vi "WHD_VEten_0.1_WS_BIDIREC_Pruebas.vi"() -> ()   [LabVIEW 2015]
uses:
  <vilib>/NI_Real-Time Target Support.lvlib
  <vilib>/rvi/interface/nirviReadWriteControl/nirviReadWriteControl.xnode
  <vilib>/rvi/interface/nirviMethod/nirviMethod.xnode
  <vilib>/rvi/interface/nirviOpenFPGA/nirviOpenFPGA.xnode
  <vilib>/rvi/interface/nirviCloseFPGA/nirviCloseFPGA.xnode
  <vilib>/userdefined/High Color/nirio_resource_hc.ctl
  <vilib>/Utility/file.llb/Write To Spreadsheet File (string).vi
  AURA_Wheel/Json2Labv.lvlib
  AURA_Wheel/AuraWheelAPI/AuraWheel.lvlib
  <vilib>/LabVIEW Targets/FPGA/cRIO/shared/nicrio_ModuleControls/nicrio_cRIO-9234_DataRatesRing2.ctl
  NiFpgaLv.dll
  <vilib>/Utility/error.llb/Error Cluster From Error Code.vi
  <vilib>/rvi/errors/niLvFpgaAdjustHostInterfaceError.vi
  <vilib>/rvi/errors/niLvFpgaMergeErrorWithErrorCode.vi
  <vilib>/Utility/file.llb/Write Delimited Spreadsheet (string).vi
  FPGA Bitfiles/W&RDEuskotrenIBA_FPGATarget2_FPGA8a2wsBIdirec_MwruJOs6jio.lvbitx
  <vilib>/FPGAPlugInAG/cRIO-9031/niLvFpga_Close_cRIO-9031.vi
  <vilib>/FPGAPlugInAG/cRIO-9031/niLvFpga_Open_cRIO-9031.vi
  <vilib>/FPGAPlugInAG/cRIO-9031/niLvFpga_Run_cRIO-9031.vi
  <vilib>/FPGAPlugInAG/cRIO-9031/niLvFpga_ConfigureFifo_cRIO-9031.vi
  <vilib>/FPGAPlugInAG/cRIO-9031/niLvFpga_StartFifo_cRIO-9031.vi
  <vilib>/FPGAPlugInAG/cRIO-9031/niLvFpga_ReadFifo_cRIO-9031.vi
  <vilib>/FPGAPlugInAG/cRIO-9031/niLvFpga_StopFifo_cRIO-9031.vi
  <vilib>/FPGAPlugInAG/cRIO-9031/niLvFpga_Reset_cRIO-9031.vi
panel:
  out "TAGs_AURAwheel":string[][](array[string])
  out "Plataformas?":bool
  out "Ejes_convoy":i32
  out "Nº Ejes":i32[](array[numeric])
  out "Nº UTs":i32
  out "it-read-LR6":i32[](array[numeric])
  out "it-LR6":i32
  out "RFID_LR6_Error":errorcluster
  out "TAGs HEX":string[](array[string])
  out "TAGs LR6":string[](array[string])
  in  "TAGs HEX 2":string[](array[string])
  out "Series_flota":string[](array[string])
  out "Tabla_flota":string[][](array[string])
  out "Puntos medios de las ventanas":dbl[][](array[numeric])
  in  "User":string
  in  "Índice de los archivos seleccionados":i32
  in  "Array":path[][](array[path])=[[path "c:/Trenes_prueba/0207_2013-09-24_19-09-42_0.bin", path "c:/Trenes_prueba/0096_2013-10-30_18-13-14_0.bin", path "c:/Trenes_prueba/0001_2013-06-05_13-06-23_0.bin"], [path "c:/Trenes_prueba/0207_2013-09-24_19-09-42_1.bin", path "c:/Trenes_prueba/0096_2013-10-30_18-13-14_1.bin", path "c:/Trenes_prueba/0001_2013-06-05_13-06-23_1.bin"], [path "c:/Trenes_prueba/0207_2013-09-24_19-09-42_2.bin", path "c:/Trenes_prueba/0096_2013-10-30_18-13-14_2.bin", path "c:/Trenes_prueba/0001_2013-06-05_13-06-23_2.bin"], [path "c:/Trenes_prueba/0207_2013-09-24_19-09-42_3.bin", path "c:/Trenes_prueba/0096_2013-10-30_18-13-14_3.bin", path "c:/Trenes_prueba/0001_2013-06-05_13-06-23_3.bin"], [path "c:/Trenes_prueba/0207_2013-09-24_19-09-42_4.bin", path "c:/Trenes_prueba/0096_2013-10-30_18-13-14_4.bin", path "c:/Trenes_prueba/0001_2013-06-05_13-06-23_4.bin"], [path "c:/Trenes_prueba/0207_2013-09-24_19-09-42_5.bin", path "c:/Trenes_prueba/0096_2013-10-30_18-13-14_5.bin", path "c:/Trenes_prueba/0001_2013-06-05_13-06-23_5.bin"], [path "c:/Trenes_prueba/0207_2013-09-24_19-09-42_6.bin", path "c:/Trenes_prueba/0096_2013-10-30_18-13-14_6.bin", path "c:/Trenes_prueba/0001_2013-06-05_13-06-23_6.bin"], [path "c:/Trenes_prueba/0207_2013-09-24_19-09-42_7.bin", path "c:/Trenes_prueba/0096_2013-10-30_18-13-14_7.bin", path "c:/Trenes_prueba/0001_2013-06-05_13-06-23_7.bin"], [path "c:/Trenes_prueba/0207_2013-09-24_19-09-42_8.bin", path "c:/Trenes_prueba/0096_2013-10-30_18-13-14_8.bin", path "c:/Trenes_prueba/0001_2013-06-05_13-06-23_8.bin"]]
  out "configuration file path":path=path "c:/Parametros.cfg"
  in  "IP synchr":string
  in  "Canal ccero?":bool
  in  "Digital?":bool=TRUE
  out "Numeric 3":i32
  out "data":cluster{"status":string}
  out "confRFID":path=path "c:/RFID/TAGS.csv"
  out "TAGS leidos":path=path "c:/RFID/TAGS.csv"
  in  "Use Aura?":bool
  in  "Parametros AuraWheel":string[](array[string])
  in  "Parámetros acelerómetros":dbl[](array[numeric])
  in  "Number of Samples":u32=5000
  in  "x*y":dbl[](array[numeric])=array[252000 elements]
  out "RFID_Error 2":errorcluster
  in  "milliseconds to wait":u32=180000
  in  "Adquirir continuado":bool
  in  "Tiempo de adquisicion":dbl=10.0
  in  "Adquirir":bool
  in  "Señal digital?":bool=TRUE
  out "Inductivo OK?":bool=TRUE
  out "Acelerómetros OK?":bool[](array[boolean])
  out "Fin":bool
  out "Contador":i32=1
  out "Path TEST":path=path "c:/TEST"
  out "Fallo fotocelula":bool
  out "Path_Borrar":path=path "c:/Trenes"
  out "Longitud de la unidad":dbl
  out "Bucle Espera":i32
  out "Aviso no detección":string
  out "Time to Acquire Block (ms)":i32
  out "Distancia de acelerómetros":dbl[](array[numeric])
  out "Block Size":u32
  out "Distancias generales":dbl[](array[numeric])
  in  "Reset del controlador":bool
  in  "Configuración":bool
  in  "Parar la aplicación":bool
  out "Acel 4":bool=TRUE
  out "Acel 3":bool=TRUE
  out "Acel 2":bool=TRUE
  out "Acel 1":bool=TRUE
  out "RFID":bool=TRUE
  out "date/time string":string
  out "Obstruido?":bool
  out "Tiempo":dbl
  out "Inicio pasada":timestamp
  out "Ultimo TEST":timestamp
  out "Fuente":bool=TRUE
  out "Estado":string
  out "RFID_ID":refnum<k5>
  out "DC OK":string
  out "Aviso temperatura":string
  in  "Tab Control":T1(tab)=enum."Parámetros"
  out "V (m/s)":dbl
  out "Temperatura (ºC)":dbl
  out "Max RMS Ruedas":dbl[][](array[numeric])
  out "result":bool
  out "TAGs":string[](array[string])
  out "Direccion 0?":bool
  out "RuedaDetectada2?":bool=TRUE
  out "RuedaDetectada1?":bool=TRUE
  out "Parar":bool
  out "Waveform Graph":sgl[][](graph)
  out "Nombre de archivo":path[](array[path])
  out "Tiempo de paso (s)":dbl
  out "Tiempo extra de adquisición (s)":dbl
  out "Número de ejes detectados":i32
  out "Buffer Underflow":bool
  out "Buffer Overflow":bool
  out "Disco Duro Disponible (bytes)":i64
  out "created path":path
  out "Nº Ruedas 1":i32
  out "NºRuedas 2":i32
  out "Fallo sensores":string
  out "T fuera rango":bool
  in  "Frecuencia de muestreo (Hz)":dbl=25600.0
  in  "Escaneos de la FIFO por canal":u32=1000
  in  "Tiempo extra al detector de paso (s)":dbl=1.0
  in  "Filtro digital (ms)":u16=13
  in  "dt RMS":dbl=256.0
  in  "Frecuencia de muestreo y módulo CRIO":T2=2 items=["51.200 kS/s (NI 9234)"=1, "25.600 kS/s (NI 9234)"=2, "17.067 kS/s (NI 9234)"=3, "12.800 kS/s (NI 9234)"=4, "10.240 kS/s (NI 9234)"=5, "8.533 kS/s (NI 9234)"=6, "7.314 kS/s (NI 9234)"=7, "6.400 kS/s (NI 9234)"=8, "5.689 kS/s (NI 9234)"=9, "5.120 kS/s (NI 9234)"=10, "4.654 kS/s (NI 9234)"=11, "4.267 kS/s (NI 9234)"=12, "3.938 kS/s (NI 9234)"=13, "3.657 kS/s (NI 9234)"=14, "3.413 kS/s (NI 9234)"=15, "3.200 kS/s (NI 9234)"=16, "3.012 kS/s (NI 9234)"=17, "2.845 kS/s (NI 9234)"=18, "2.695 kS/s (NI 9234)"=19, "2.560 kS/s (NI 9234)"=20, "2.438 kS/s (NI 9234)"=21, "2.328 kS/s (NI 9234)"=22, "2.226 kS/s (NI 9234)"=23, "2.133 kS/s (NI 9234)"=24, "2.048 kS/s (NI 9234)"=25, "1.969 kS/s (NI 9234)"=26, "1.896 kS/s (NI 9234)"=27, "1.829 kS/s (NI 9234)"=28, "1.765 kS/s (NI 9234)"=29, "1.707 kS/s (NI 9234)"=30, "1.652 kS/s (NI 9234)"=31]
  in  "Puerto RFID":u16=2189
  in  "IP RFID":string="192.168.106.99"
  in  "Offset_rueda":fxp<+/-,24,-4>=0.004999998956918716 format="%.27g"
  in  "Count(mSec)":u32=2
  in  "LR6 IP address":string="192.168.106.94"
  in  "Port LR6":u16=2001
  in  "Number of Channels":u32=9
  in  "Pruebas RFID 2":bool
  in  "Pruebas RFID 1":bool
  in  "Descargar":bool
  out "Parámetros":bool=TRUE
  out "Distacias y medidas de dispositivos":bool=TRUE
  out "RFID_Error":errorcluster
  out "error FPGA":errorcluster
  out "error manipulacion archivos":errorcluster
  out "Unidades y ejes":bool=TRUE
  out "RFID":bool=TRUE
  out "error AURA":errorcluster
  out "Response headers":string
  # "Funciona?"
  # "Inductivo"
  # "A4"
  # "A3"
  # "A1"
  # "A2"
  # "WRD_MEX\nWRD_ZAR"
  # "0 tagMexInit\n1 tagMexFin\n\n0 tag1\n1 tag2"
  # "Última detección de unidad"
  # "Error!!"
  # "Estado de la memoria"
  # "Espera"
  # "Adquisicion"
  # "Adquisicion"
  # "Procesado"
  # "Procesado"
  # "Procesado"
  # "Procesado"
  # "Procesado"
  # "Parámetros de muestreo"
  # "Parámetros de adquisición"
  # "Parámetros de procesado"
  # "Cambio Fecha y Hora"
  # "Descarga de planos y TEST"
  # "NO"
  # "SI"
  # "Descarga archivos binarios de adquisición"
  # "NO"
  # "SI"
  # "Cargar datos de configuración"
  # "Errores!!"
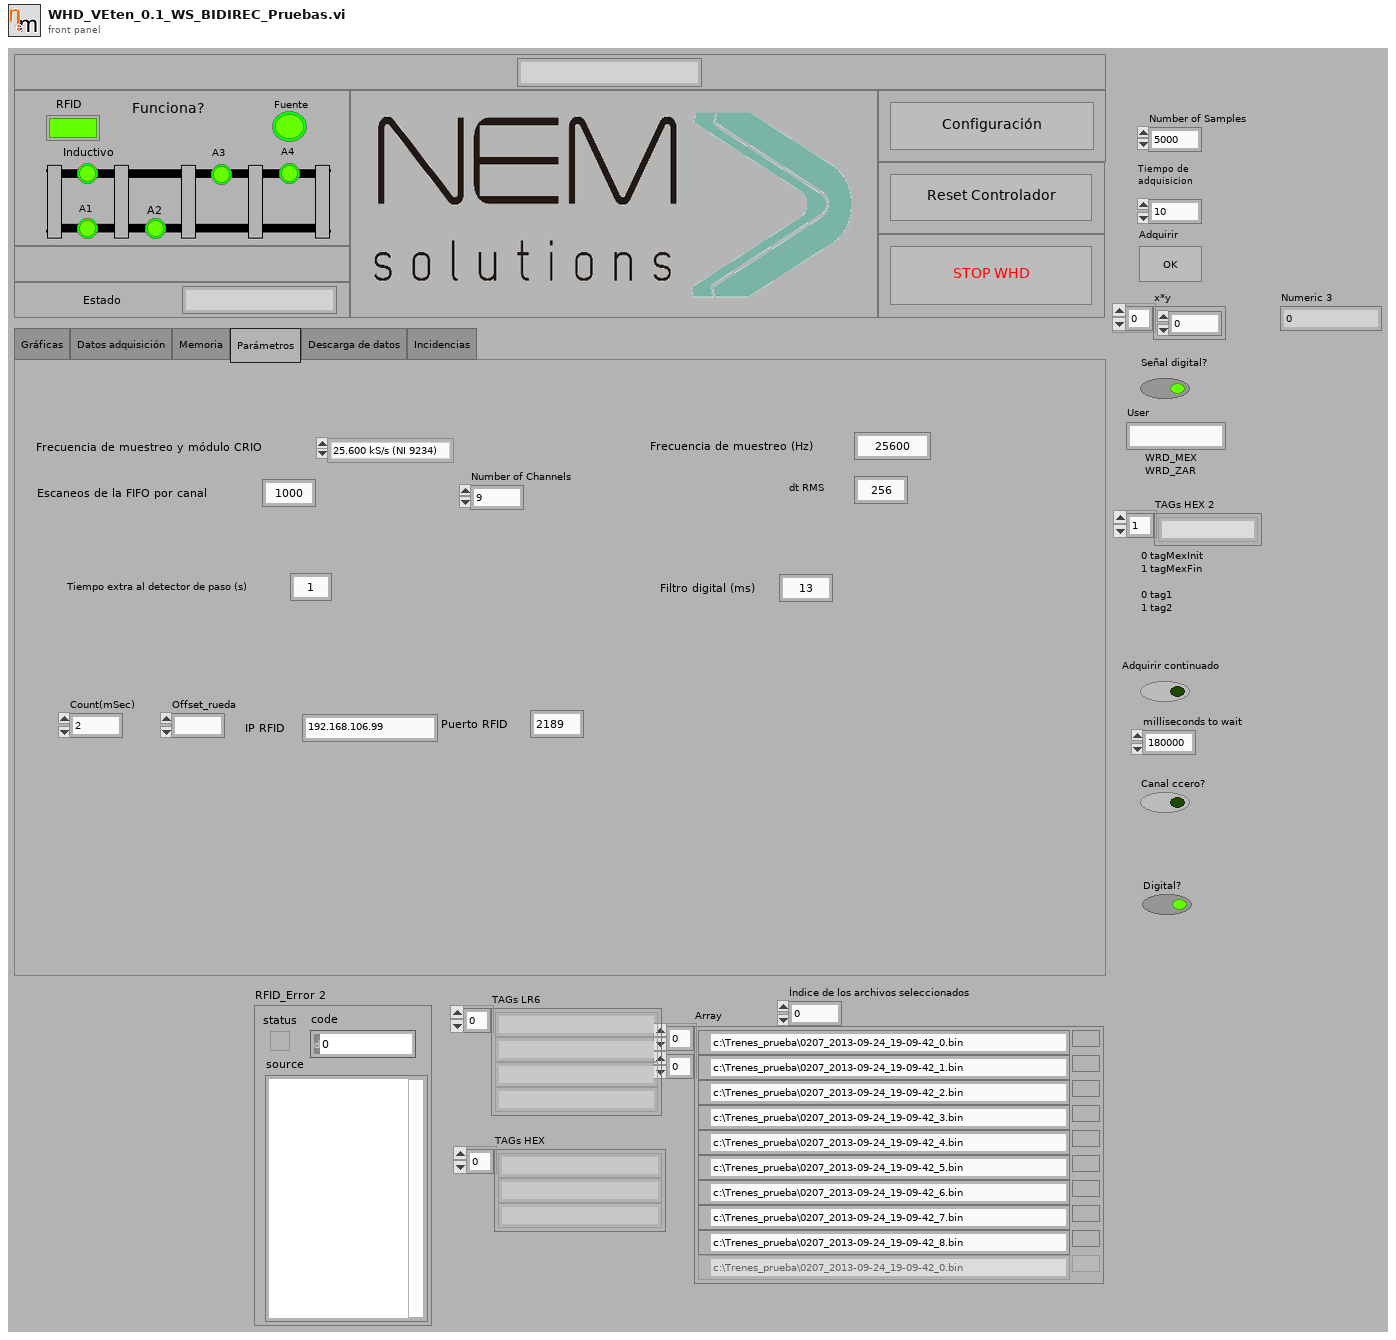
[diagram p1: front panel]
types:
  T1 = enum32{"Gráficas", "Datos adquisición", "Memoria", "Parámetros", "Descarga de datos", "Incidencias"}
  T2 = typedef "nicrio_cRIO-9234_DataRatesRing2.ctl" = u8
  T3 = typedef "nirio_resource_hc.ctl" = tag
  T4 = enum16{"Standard", "Buffered", "CRLF", "Immediate"}
  T5 = enum16{"open", "replace", "create", "open or create", "replace or create", "replace or create with confirmation"}
  T6 = enum16{"big-endian, network order", "native, host order", "little-endian"}
  T7 = cluster{"error IO":errorcluster, bool[], u32[], string[], dbl[]}
  T8 = cluster{"g_ts":dbl, "p_sp":dbl, "p_tp":dbl, "p_tg":cluster{"tg_n":dbl, "tg_t":string}[], "p_ax":cluster{"ax_n":dbl, "ax_sp":dbl, "ax_wh":cluster{"wh_p":dbl, "wh_a1":dbl, "wh_a2":dbl, "wh_a3":dbl, "wh_a4":dbl}[]}[]}
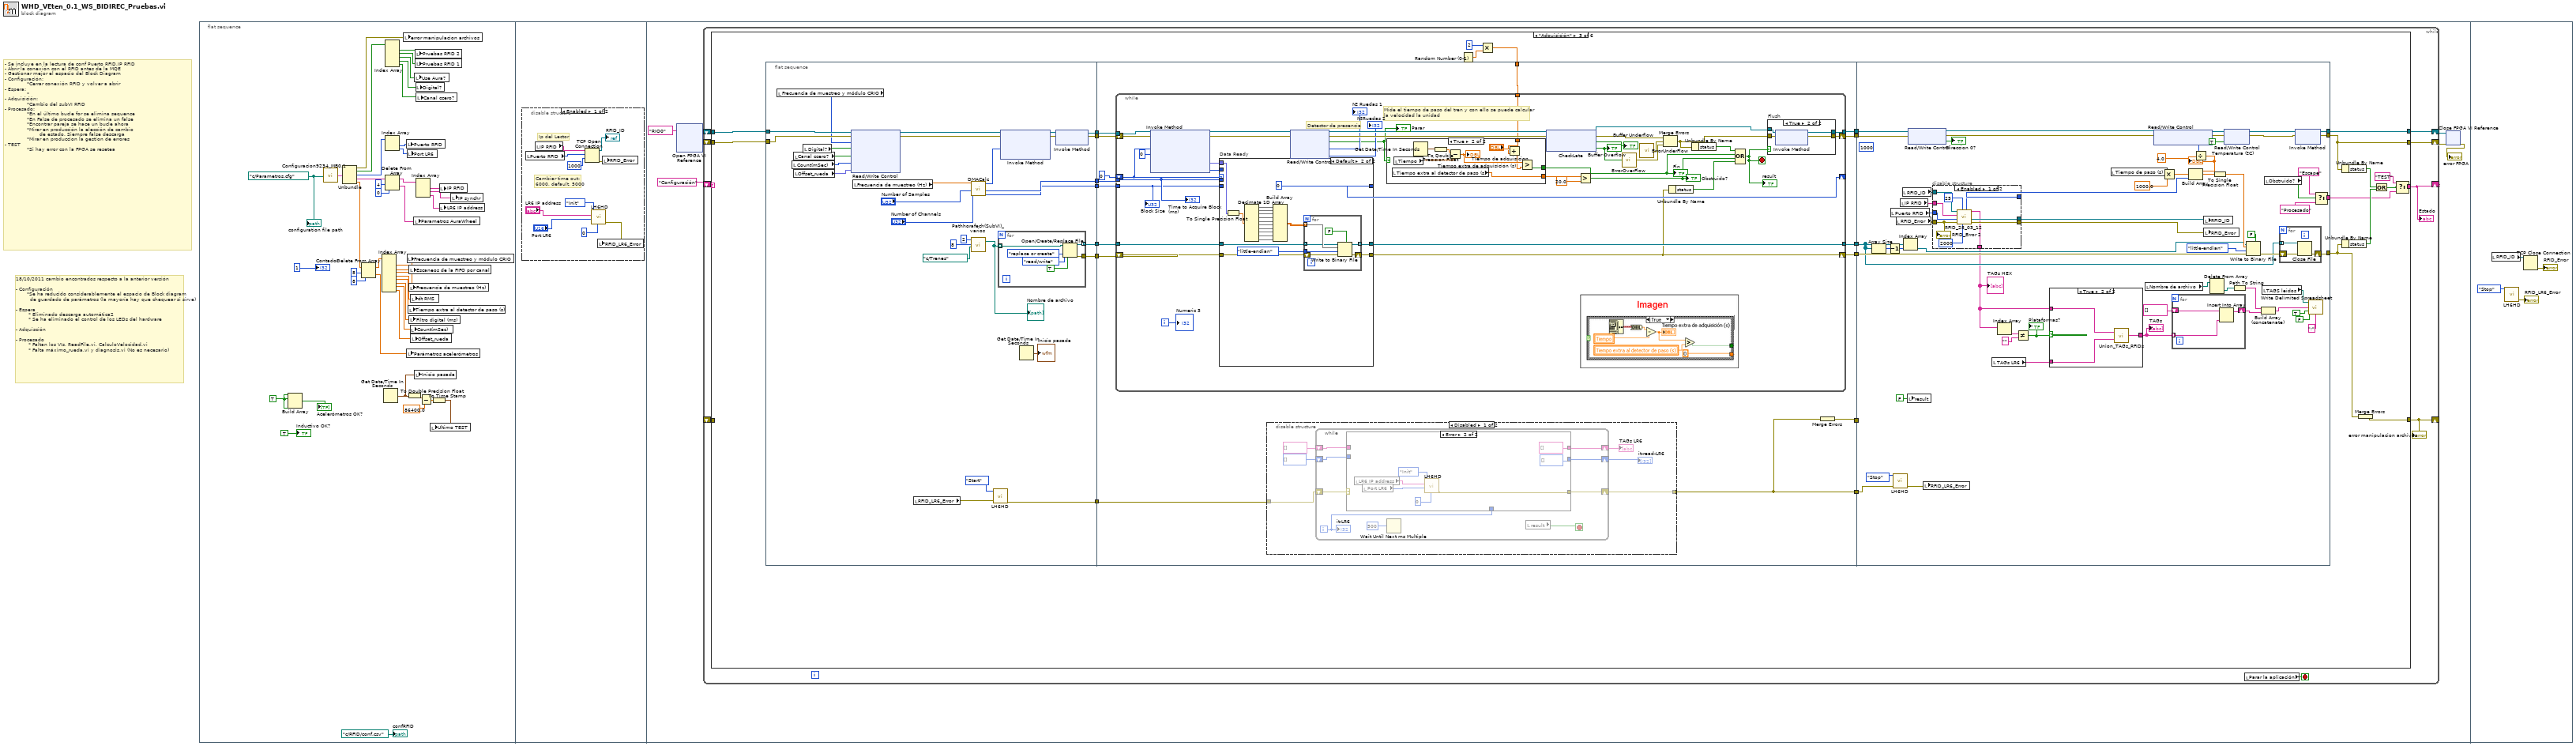
[diagram p0: block diagram]
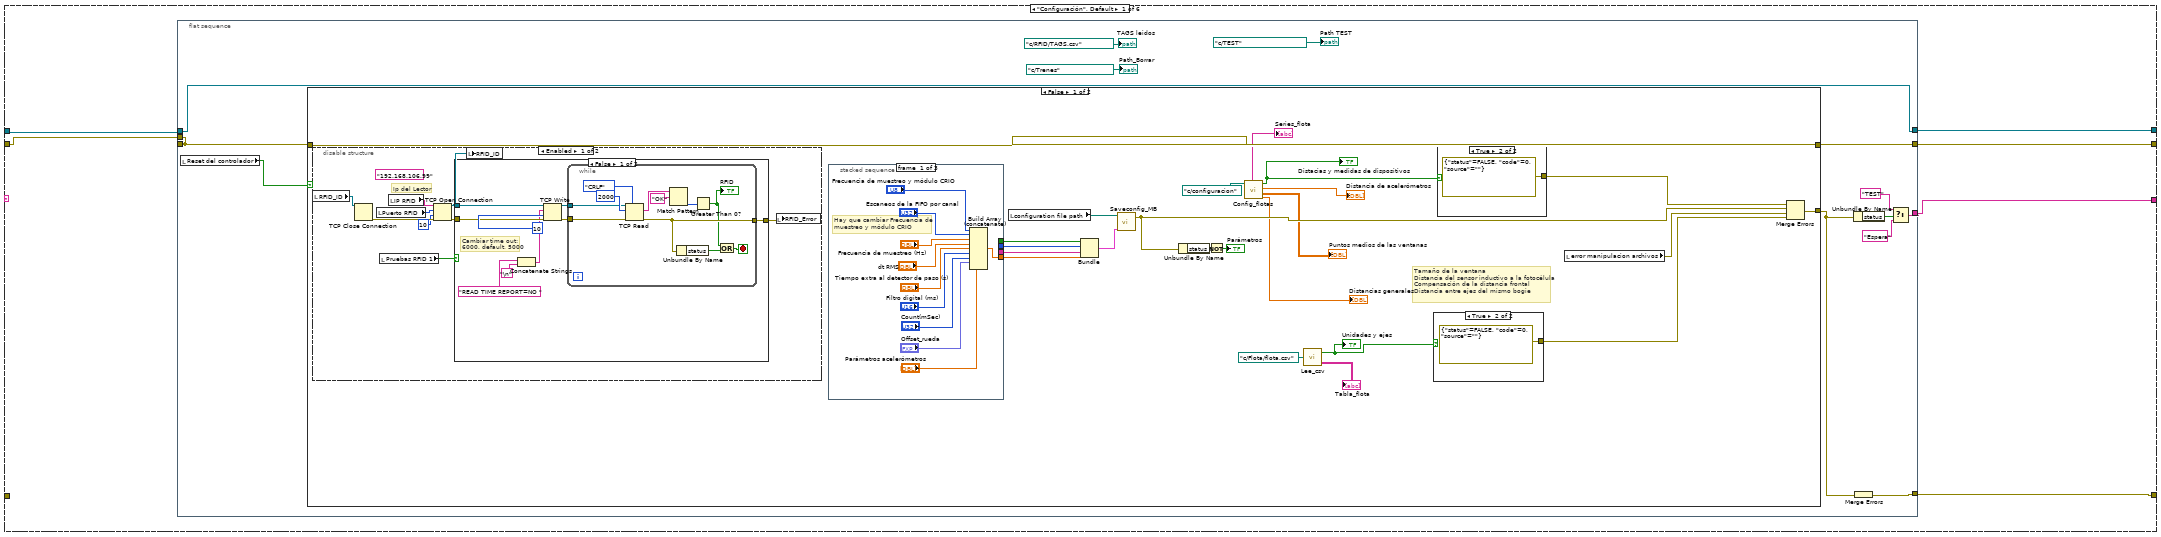
[diagram p3: hidden frame]
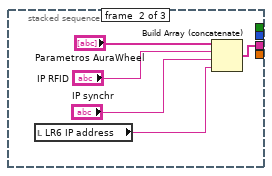
[diagram p4: hidden frame]
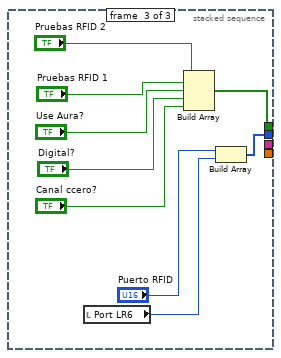
[diagram p5: hidden frame]
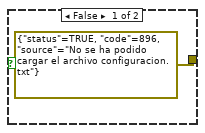
[diagram p6: hidden frame]
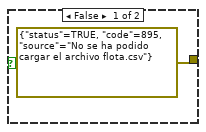
[diagram p7: hidden frame]
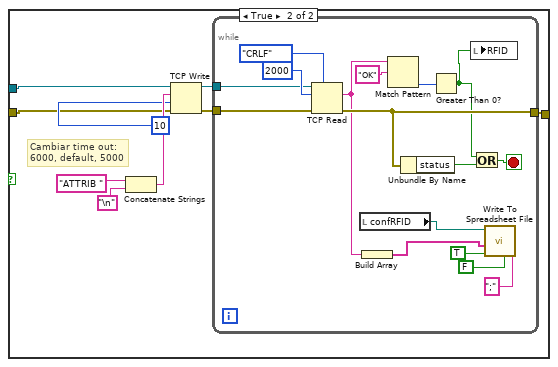
[diagram p8: hidden frame]
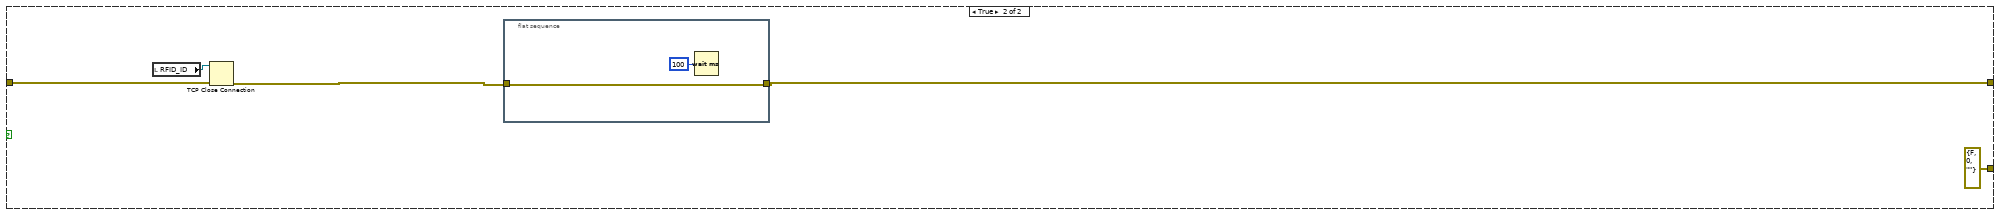
[diagram p10: hidden frame]
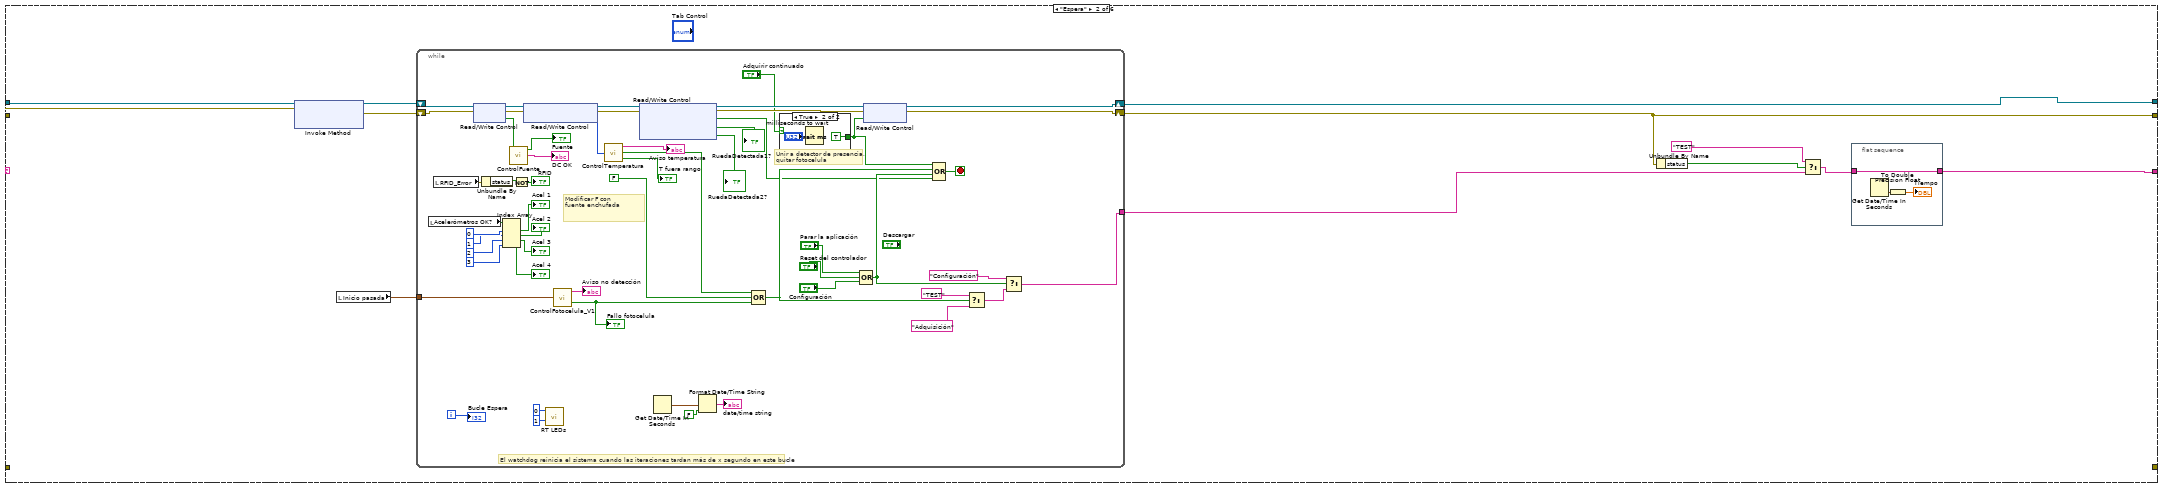
[diagram p11: hidden frame]
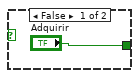
[diagram p12: hidden frame]
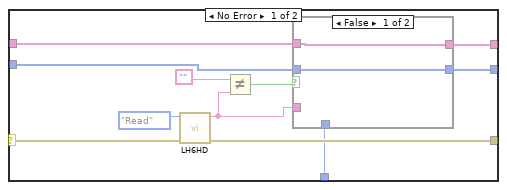
[diagram p13: hidden frame]
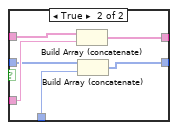
[diagram p14: hidden frame]
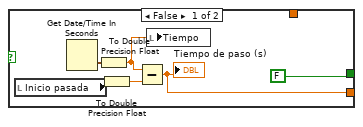
[diagram p16: hidden frame]
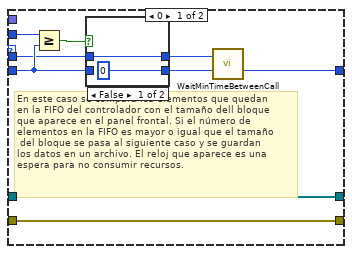
[diagram p17: hidden frame]
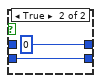
[diagram p18: hidden frame]
diagram:
  # "18/10/2011 cambio encontrados respecto a la anterior versión\n\n- Configuración\n       *Se ha reducido considerablemente el espacio de Block diagram\n         de guardado de parámetros (la mayoría hay que chequear si sirve)\n\n- Espera\n        * Eliminado descarga automática2\n        * Se ha eliminado el control de los LEDs del hardware\n       \n- Adquisción\n\n- Procesado\n        * Faltan los VIs, ReadFile.vi, CalculoVelocidad.vi\n        * Falta máximo_rueda.vi y diagnosis.vi (No es necesario)"
  # "- Se incluye en la lectura de conf Puerto RFID,IP RFID\n- Abrir la conexión con el RFID antes de la MQE\n- Gestionar mejor el espacio del Block Diagram\n- Configuración:\n              *Cerrar conexión RFID y volver a abrir\n- Espera:\n              *\n- Adquisición:\n              *Cambio del subVI RFID\n- Procesado:\n              *En el último bucle for se elimina sequence\n              *En False de procesado se elimina un false\n              *Encontrar pareja se hace un bucle ahora\n              *Mirar en producción la elección de cambio\n                      de estado. Siempre false descarga \n              *Mirar en produccion la gestion de errores\n- TEST\n              *Si hay error con la FPGA se resetea"
  n1 = flat-sequence {
    frame #0 {
      w27 = TRUE
      w23 = path "c:/Parametros.cfg" ("configuration file path")
      n2 = Build Array(w27, w27, w27, w27) -> (→"Acelerómetros OK?":bool[])
      n3 = call "Configuracion9234_MB0.1.vi"("configuration file path"=w23) -> ("output cluster"=w22:T7)
      n4 = Unbundle(w22) -> ("error IO"=w30:errorcluster, w29:bool[], w28:u32[], w14:string[], w20:dbl[])
      n5 = Delete From Array(array=w20, length=8, index=8) -> (deleted portion=w16:dbl[], array with subset deleted=w19:dbl[])
      n6 = Index Array(array=w19) -> (element #1=w38:dbl, element #2=w37:dbl, element #3=w36:dbl, element #4=w35:dbl, element #5=w34:dbl, element #6=w33:dbl, element #7=w8:dbl, element #8=w7:dbl)  [unwired: 8 in]
      n7 = Get Date/Time In Seconds() -> (seconds since 1Jan1904=w40:timestamp)
      n8 = Index Array(array=w29) -> (element #1=w32:bool, element #2=w31:bool, element #3=w15:bool, element #4=w4:bool, element #5=w9:bool)  [unwired: 5 in]
      n9 = Index Array(array=w28) -> (element #1=w21:u32, element #2=w1:u32)  [unwired: 2 in]
      n10 = Delete From Array(array=w14, length=4, index=0) -> (deleted portion=w5:string[], array with subset deleted=w13:string[])
      n11 = local write "error manipulacion archivos"(w30) -> ()
      n12 = local write "Puerto RFID"(w21) -> ()
      n13 = local write "Parámetros acelerómetros"(w16) -> ()
      n14 = local write "Port LR6"(w1) -> ()
      n15 = local write "Frecuencia de muestreo y módulo CRIO"(w38) -> ()
      n16 = To Double Precision Float(number=w40) -> (double precision float=w42:dbl)
      n17 = local write "Tiempo extra al detector de paso (s)"(w34) -> ()
      n18 = local write "Frecuencia de muestreo (Hz)"(w36) -> ()
      n19 = local write "Filtro digital (ms)"(w33) -> ()
      n20 = local write "Escaneos de la FIFO por canal"(w37) -> ()
      n21 = local write "Count(mSec)"(w8) -> ()
      n22 = local write "dt RMS"(w35) -> ()
      n23 = local write "Offset_rueda"(w7) -> ()
      n24 = local write "Parametros AuraWheel"(w5) -> ()
      n25 = local write "Inicio pasada"(w40) -> ()
      n26 = local write "Use Aura?"(w15) -> ()
      n27 = local write "Pruebas RFID 2"(w32) -> ()
      n28 = local write "Pruebas RFID 1"(w31) -> ()
      n29 = local write "Digital?"(w4) -> ()
      n30 = Index Array(array=w13) -> (element #1=w3:string, element #2=w6:string, element #3=w2:string)  [unwired: 3 in]
      n31 = local write "Canal ccero?"(w9) -> ()
      n32 = Subtract(x=w42, y=86400.0) -> (x-y=w41:dbl)
      n33 = To Time Stamp(1:w41) -> (0:w39:timestamp)
      n34 = local write "Ultimo TEST"(w39) -> ()
      n35 = local write "IP RFID"(w3) -> ()
      n36 = local write "LR6 IP address"(w2) -> ()
      n37 = local write "IP synchr"(w6) -> ()
      "Contador" <- 1
      "Inductivo OK?" <- TRUE ("Inductivo OK?")
      "confRFID" <- path "c:/RFID/conf.csv" ("file path (use dialog)")
      "configuration file path" <- w23
    }
    frame #1 {
      n38 = disable-structure shown="Enabled" {
        frame Enabled {
          # "Cambiar time out:\n6000, default, 5000"
          # "Ip del Lector"
          n39 = local read "Puerto RFID"() -> (w50:u16)
          n40 = local read "IP RFID"() -> (w51:string)
          n41 = TCP Open Connection(address=w51, remote port or service name=w50, timeout ms (60000)=1000) -> (connection ID=→"RFID_ID":refnum<k5>, error out=w49:errorcluster)  [unwired: 1 in, 1 out]
          n42 = call "LH6HD.vi"("DeviceAddress"=u8 0, "Reader Port"="Port LR6", "IP Address"="LR6 IP address", "Action"=enum16{"Init", "Start", "Read", "Stop", "Exit"}."Init") -> ("error out"=w48:errorcluster)  [unwired: 6 in, 1 out]
          n43 = local write "RFID_LR6_Error"(w48) -> ()
          n44 = local write "RFID_Error"(w49) -> ()
        }
        frame Disabled {
        }
      }
    }
    frame #2 {
      n45 = xnode "Open FPGA VI Reference"("resource name"=T3 "RIO0") -> ("FPGA VI Reference Out"=w60:refnum<k20>, "error out"=w59:errorcluster)  [unwired: 1 in]
      n46 = while {
        shift-right: [w64] -> _
        shift-left: "Configuración" -> [w69]
        shift-right: [w62] -> w56
        shift-left: w60 -> [w68]
        shift-right: [w61] -> w55
        shift-left: w59 -> [w67]
        shift-right: [w66] -> _
        shift-left: _ -> [w65]
        stop <- w63 stop-if-true
        n47 = case shown="\"Adquisición\"" w69 {
          tunnel: [w74 w201 w279 w579 w791 "TEST" ("t")] -> w64
          tunnel: [w73 w203 w293 w587 w789 w853] -> w62
          tunnel: [w75 w202 w294 w574 w786 w850] -> w61
          tunnel: w68 -> [w72 w208 w301 w587 w789 w852]
          tunnel: w67 -> [w71 w206 w300 w574 w788 w849]
          tunnel: [w70 _ w291 w577 w787 w854] -> w66
          tunnel: w65 -> [_ _ _ w572 w790 w854]
          frame "Configuración", Default {
            n48 = flat-sequence {
              tunnel: [w77] -> _
              tunnel: [w79] -> w75
              tunnel: [w87] -> w74
              tunnel: w72 -> [w80]
              tunnel: [w80] -> w73
              tunnel: [w82] -> w70
              tunnel: w71 -> [w77]
              frame #0 {
                n49 = local read "Reset del controlador"() -> (w76:bool)
                n50 = case shown="False" w76 {
                  tunnel: w77 -> [w111 w196]
                  tunnel: [w111 w195] -> w79
                  tunnel: [w97 errorcluster {"status"=FALSE, "code"=0, "source"=""} ("error IO")] -> w78
                  frame False {
                    # "Tamaño de la ventana\nDistancia del sensor inductivo a la fotocélula\nCompensación de la distancia frontal\nDistancia entre ejes del mismo bogie"
                    n51 = disable-structure shown="Enabled" {
                      frame Enabled {
                        (unwired) "192.168.106.99" ("address")
                        # "Ip del Lector"
                        n52 = local read "RFID_ID"() -> (w147:refnum<k5>)
                        n53 = TCP Close Connection(connection ID=w147) -> (error out=w148:errorcluster)  [unwired: 2 in, 1 out]
                        n54 = local read "Puerto RFID"() -> (w145:u16)
                        n55 = local read "Pruebas RFID 1"() -> (w140:bool)
                        n56 = local read "IP RFID"() -> (w144:string)
                        n57 = TCP Open Connection(address=w144, remote port or service name=w145, timeout ms (60000)=10, error in (no error)=w148) -> (connection ID=w146:refnum<k5>, error out=w141:errorcluster)  [unwired: 1 out]
                        n58 = case shown="False" w140 {
                          tunnel: w146 -> [w157 w171]
                          tunnel: [w155 w169] -> w142
                          tunnel: w141 -> [w152 w170]
                          frame False {
                            # "Cambiar time out:\n6000, default, 5000"
                            n59 = Concatenate Strings("READ TIME REPORT=NO " ("data in"), "\n") -> (w149:string)
                            n60 = TCP Write(connection ID=w157, data in=w149, error in (no error)=w152, 9:10 ("timeout ms (25000)")) -> (connection ID out=w153:refnum<k5>, error out=w154:errorcluster)  [unwired: 1 out]
                            n61 = while {
                              tunnel: w154 -> [w166]
                              tunnel: w153 -> [w165]
                              tunnel: [w164] -> w155
                              stop <- w161 stop-if-true
                              n62 = TCP Read(connection ID=w165, bytes to read=2000, error in (no error)=w166, 7:T4."CRLF" ("mode (standard)")) -> (data out=w159:string, error out=w164:errorcluster)  [unwired: 1 in, 1 out]
                              n63 = Match Pattern(string=w159, regular expression="OK") -> (offset past match=w162:i32)  [unwired: 4 out]
                              n64 = Unbundle By Name(w164) -> ("status"=w160:bool)
                              n65 = Greater Than 0?(x=w162) -> (x > 0?=w158:bool)
                              "RFID" <- w158
                              n66 = Or(x=w158, y=w160) -> (x .or. y?=w161:bool)
                            }
                          }
                          frame True {
                            # "Cambiar time out:\n6000, default, 5000"
                            n67 = Concatenate Strings("ATTRIB " ("data in"), "\n") -> (w177:string)
                            n68 = TCP Write(connection ID=w171, data in=w177, error in (no error)=w170, 9:10 ("timeout ms (25000)")) -> (connection ID out=w174:refnum<k5>, error out=w173:errorcluster)  [unwired: 1 out]
                            n69 = while {
                              tunnel: w173 -> [w191]
                              tunnel: w174 -> [w190]
                              tunnel: [w189] -> w169
                              stop <- w186 stop-if-true
                              n70 = TCP Read(connection ID=w190, bytes to read=2000, error in (no error)=w191, 7:T4."CRLF" ("mode (standard)")) -> (data out=w180:string, error out=w189:errorcluster)  [unwired: 1 in, 1 out]
                              n71 = local read "confRFID"() -> (w178:path)
                              n72 = Build Array(w180) -> (w179:string[])
                              n73 = Match Pattern(string=w180, regular expression="OK") -> (offset past match=w187:i32)  [unwired: 4 out]
                              n74 = Unbundle By Name(w189) -> ("status"=w185:bool)
                              n75 = Greater Than 0?(x=w187) -> (x > 0?=w184:bool)
                              n76 = local write "RFID"(w184) -> ()
                              n77 = Or(x=w184, y=w185) -> (x .or. y?=w186:bool)
                              n78 = call-poly <vilib>:"Write To Spreadsheet File.vi"("delimiter (\\t)"=";" ("delimiter (\\t)"), "transpose? (no:F)"=FALSE, "append to file? (new file:F)"=TRUE, "1D data"=w179, "file path (dialog if empty)"=w178) -> ()  [unwired: 3 in, 1 out]
                            }
                          }
                        }
                        n79 = local write "RFID_ID"(w146) -> ()
                        n80 = local write "RFID_Error"(w142) -> ()
                      }
                      frame Disabled {
                      }
                    }
                    n81 = stacked-sequence {
                      tunnel: [w116 _ _] -> w101
                      tunnel: [_ w126 _] -> w100
                      tunnel: [_ _ w132] -> w102
                      tunnel: [_ _ w131] -> w103
                      frame #0 {
                        # "Hay que cambiar Frecuencia de\nmuestreo y módulo CRIO"
                        n82 = Build Array (concatenate)("Frecuencia de muestreo y módulo CRIO", "Escaneos de la FIFO por canal", "Frecuencia de muestreo (Hz)", "dt RMS", "Tiempo extra al detector de paso (s)", "Filtro digital (ms)", "Count(mSec)", "Offset_rueda", "Parámetros acelerómetros") -> (w116:dbl[])
                      }
                      frame #1 {
                        n83 = local read "LR6 IP address"() -> (w122:string)
                        n84 = Build Array (concatenate)("Parametros AuraWheel", "IP RFID", "IP synchr", w122) -> (w126:string[])
                      }
                      frame #2 {
                        n85 = local read "Port LR6"() -> (w127:u16)
                        n86 = Build Array("Pruebas RFID 2", "Pruebas RFID 1", "Use Aura?", "Digital?", "Canal ccero?") -> (w131:bool[])
                        n87 = Build Array("Puerto RFID", w127) -> (w132:u16[])
                      }
                    }
                    n88 = local read "configuration file path"() -> (w98:path)
                    n89 = Bundle(w103, w102, w100, w101) -> (w99:cluster{bool[], u16[], string[], dbl[]})  [unwired: 1 in]
                    n90 = call "Saveconfig_MB.vi"("configuration file path"=w98, "Configuracion"=w99) -> ("error out"=w106:errorcluster)  [unwired: 4 in]
                    n91 = Unbundle By Name(w106) -> ("status"=w107:bool)
                    n92 = Not(x=w107) -> (.not. x?=→"Parámetros":bool)
                    n93 = call "Config_flotas.vi"("file path (dialog if empty)"=path "c:/configuracion") -> ("Distancias generales"=→"Distancias generales":dbl[], "Puntos medios de las ventanas"=→"Puntos medios de las ventanas":dbl[][], "Distancia de acelerómetros"=→"Distancia de acelerómetros":dbl[], "Distacias y medidas de dispositivos"=w96:bool, "Series_flota"=→"Series_flota":string[])  [unwired: 3 in]
                    "Distacias y medidas de dispositivos" <- w96
                    n94 = call "Lee_csv.vi"("Path"=path "c:/Flota/flota.csv") -> ("Tabla_flota"=→"Tabla_flota":string[][], "Lectura_OK?"=w92:bool)
                    "Unidades y ejes" <- w92
                    n95 = case shown="True" w92 {
                      tunnel: [errorcluster {"status"=TRUE, "code"=895, "source"="No se ha podido cargar el archivo flota.csv"} ("error out") errorcluster {"status"=FALSE, "code"=0, "source"=""} ("error out")] -> w104
                      frame False {
                      }
                      frame True {
                      }
                    }
                    n96 = case shown="True" w96 {
                      tunnel: [errorcluster {"status"=TRUE, "code"=896, "source"="No se ha podido cargar el archivo configuracion.txt"} ("error out") errorcluster {"status"=FALSE, "code"=0, "source"=""} ("error out")] -> w109
                      frame False {
                      }
                      frame True {
                      }
                    }
                    n97 = local read "error manipulacion archivos"() -> (w105:errorcluster)
                    n98 = Merge Errors(w109, w106, w105, w104) -> (w97:errorcluster)
                  }
                  frame True {
                    n99 = local read "RFID_ID"() -> (w198:refnum<k5>)
                    n100 = TCP Close Connection(connection ID=w198, error in (no error)=w196) -> (error out=w194:errorcluster)  [unwired: 2 out]
                    n101 = flat-sequence {
                      tunnel: [w200] -> w195
                      tunnel: w194 -> [w200]
                      frame #0 {
                        n102 = Wait (ms)(milliseconds to wait=u32 100) -> ()  [unwired: 1 out]
                      }
                    }
                  }
                }
                n103 = Unbundle By Name(w78) -> ("status"=w88:bool)
                n104 = Merge Errors(w78) -> (w82:errorcluster)
                n105 = Select(t="TEST", s=w88, f="Espera") -> (s? t:f=w87:string)
                "Path_Borrar" <- path "c:/Trenes" ("file path (use dialog)")
                "Path TEST" <- path "c:/TEST" ("file path (use dialog)")
                "TAGS leidos" <- path "c:/RFID/TAGS.csv" ("file path (use dialog)")
              }
            }
          }
          frame "Espera" {
            n106 = xnode "Invoke Method"("FPGA VI Reference In"=w208, "error in"=w206) -> ("FPGA VI Reference Out"=w207:refnum<k20>, "error out"=w205:errorcluster)  [unwired: 1 in]
            n107 = local read "Inicio pasada"() -> (w212:timestamp)
            n108 = while {
              tunnel: [w229] -> w211
              shift-right: [w217] -> w203
              shift-left: w207 -> [w231]
              shift-right: [w216] -> w202
              shift-left: w205 -> [w230]
              tunnel: w212 -> [w240]
              i -> [w263]
              stop <- w270 stop-if-true
              # "Modificar F con\nfuente enchufada"
              # "Unir a detector de presencia,\nquitar fotocelula"
              # "El watchdog reinicia el sistema cuando las iteraciones tardan más de x segundo en este bucle"
              n109 = local read "Acelerómetros OK?"() -> (w239:bool[])
              n110 = local read "RFID_Error"() -> (w247:errorcluster)
              n111 = xnode "Read/Write Control"("FPGA VI Reference In"=w231, "error in"=w230) -> ("FPGA VI Reference Out"=w258:refnum<k20>, "error out"=w257:errorcluster, "DC OK"=w262:bool)
              n112 = Unbundle By Name(w247) -> ("status"=w245:bool)
              n113 = Index Array(array=w239, index #1=0 ("index"), index #2=1 ("index"), index #3=2 ("index"), index #4=3 ("index")) -> (element #1=→"Acel 1":bool, element #2=→"Acel 2":bool, element #3=→"Acel 3":bool, element #4=→"Acel 4":bool)
              n114 = call "ControlFuente.vi"("DC OK 3"=w262) -> ("DC OK 2"=→"Fuente":bool, "DC OK"=→"DC OK":string)  [unwired: 1 out]
              n115 = Not(x=w245) -> (.not. x?=→"RFID":bool)
              n116 = xnode "Read/Write Control"("FPGA VI Reference In"=w258, "error in"=w257) -> ("FPGA VI Reference Out"=w253:refnum<k20>, "error out"=w252:errorcluster, "Chassis Temperature"=w260:i16)
              n117 = call <vilib>:"RT LEDs.vi"("State"=1, "LED Num"=0) -> ()  [unwired: 1 in, 5 out]
              n118 = call "ControlFotocelula_V1.vi"("Tiempo de entrada a espera"=w240) -> ("Aviso no detección"=→"Aviso no detección":string, "Boolean"=w250:bool)
              "Fallo fotocelula" <- w250
              n119 = call "ControlTemperatura.vi"("Chassis Temperature"=w260) -> ("Aviso temperatura"=→"Aviso temperatura":string, "Boolean"=w254:bool, "T fuera rango"=→"T fuera rango":bool)
              n120 = xnode "Read/Write Control"("FPGA VI Reference In"=w253, "error in"=w252) -> ("FPGA VI Reference Out"=w234:refnum<k20>, "error out"=w233:errorcluster, "Detector de presencia"=w224:bool, "RuedaDetectada1?"=→"RuedaDetectada1?":bool, "RuedaDetectada2?"=→"RuedaDetectada2?":bool)
              n121 = Get Date/Time In Seconds() -> (seconds since 1Jan1904=w226:timestamp)
              n122 = Format Date/Time String(seconds (now)=w226, UTC format=FALSE) -> (date/time string=→"date/time string":string)  [unwired: 1 in]
              n123 = Compound Arithmetic op=OR(w254, FALSE ("value"), w250) -> (w251:bool)
              n124 = case shown="True" "Adquirir continuado" {
                tunnel: ["Adquirir" TRUE ("Adquirir")] -> w228
                frame False {
                }
                frame True {
                  n125 = Wait (ms)(milliseconds to wait="milliseconds to wait") -> ()  [unwired: 1 out]
                }
              }
              n126 = Compound Arithmetic op=OR("Parar la aplicación", "Reset del controlador", "Configuración") -> (w248:bool)
              n127 = xnode "Read/Write Control"("FPGA VI Reference In"=w234, "error in"=w233, "Fotocélula"=w228) -> ("FPGA VI Reference Out"=w217:refnum<k20>, "error out"=w216:errorcluster)
              n128 = Compound Arithmetic op=OR(w228, w251, w248, w224) -> (w270:bool)
              n129 = Select(t="TEST", s=w251, f="Adquisición") -> (s? t:f=w266:string)
              n130 = Select(t="Configuración", s=w248, f=w266) -> (s? t:f=w229:string)
              "Bucle Espera" <- w263
            }
            n131 = Unbundle By Name(w202) -> ("status"=w210:bool)
            n132 = Select(t="TEST", s=w210, f=w211) -> (s? t:f=w204:string)
            n133 = flat-sequence {
              tunnel: [w214] -> w201
              tunnel: w204 -> [w214]
              frame #0 {
                n134 = Get Date/Time In Seconds() -> (seconds since 1Jan1904=w215:timestamp)
                n135 = To Double Precision Float(number=w215) -> (double precision float=→"Tiempo":dbl)
              }
            }
          }
          frame "Adquisición" {
            n136 = flat-sequence {
              tunnel: w300 -> [w325]
              tunnel: w301 -> [w326]
              tunnel: [w324] -> w290
              tunnel: [w323] -> w289
              tunnel: [w322] -> w288
              tunnel: [w321] -> w287
              tunnel: [w320] -> w286
              tunnel: [w319] -> w285
              tunnel: [w302] -> w275
              tunnel: [w339] -> w299
              tunnel: [w351] -> w298
              tunnel: [w350] -> w297
              tunnel: [w349] -> w296
              tunnel: [w342] -> w295
              tunnel: w290 -> [w348]
              tunnel: w289 -> [w347]
              tunnel: w288 -> [w346]
              tunnel: w287 -> [w345]
              tunnel: w286 -> [w344]
              tunnel: w285 -> [w343]
              tunnel: w276 -> [w341]
              tunnel: w275 -> [w338]
              tunnel: [w337] -> w274
              tunnel: w299 -> [_]
              tunnel: w298 -> [w495]
              tunnel: w297 -> [w494]
              tunnel: w296 -> [w510]
              tunnel: [w540] -> w282
              tunnel: w295 -> [w542]
              tunnel: [w526] -> w292
              tunnel: [w527] -> w294
              tunnel: [w528] -> w293
              tunnel: w274 -> [w503]
              frame #0 {
                n137 = local read "Frecuencia de muestreo y módulo CRIO"() -> (w309:T2)
                n138 = local read "Count(mSec)"() -> (w306:u32)
                n139 = local read "Canal ccero?"() -> (w307:bool)
                n140 = local read "Offset_rueda"() -> (w305:fxp<+/-,24,-4>)
                n141 = local read "Digital?"() -> (w308:bool)
                n142 = xnode "Read/Write Control"("FPGA VI Reference In"=w326, "error in"=w325, "Data Rate"=w309, "Digital?"=w308, "Canal cero WS1?"=w307, "Count(mSec)"=w306, "Offset_rueda"=w305) -> ("FPGA VI Reference Out"=w315:refnum<k20>, "error out"=w314:errorcluster)
                n143 = local read "Frecuencia de muestreo (Hz)"() -> (w317:dbl)
                n144 = local read "RFID_LR6_Error"() -> (w303:errorcluster)
                n145 = call "DMACalc.vi"("Number of Channels"="Number of Channels", "Number of Samples"="Number of Samples", "Rate (Hz)"=w317) -> ("Block Size"=w321:u32, "Time to Acquire Block (ms)"=w322:i32, "Host Buffer Size"=w327:u32)  [unwired: 6 in]
                n146 = call "Pathhorafech(SubVI)_varios.vi"("Folder path"=path "c:/Trenes", "Nº de acelerómetros"=8, "Nº inductivos"=2) -> ("Acel_Paths"=w310:path[])  [unwired: 1 in, 1 out]
                "Nombre de archivo" <- w310
                n147 = call "LH6HD.vi"("error in (no error)"=w303, "Action"=enum16{"Init", "Start", "Read", "Stop", "Exit"}."Start") -> ("error out"=w302:errorcluster)  [unwired: 8 in, 1 out]
                n148 = for {
                  tunnel: w310 -> [w333] mode=indexing
                  tunnel: [w332] -> w320 mode=indexing
                  tunnel: [w331] -> w319
                  n149 = Open/Create/Replace File(file path (use dialog)=w333, operation (0:open)=T5."replace or create", access (0:read/write)=enum16{"read/write", "read-only", "write-only"}."read/write", disable buffering (F)=TRUE) -> (refnum out=w332:refnum<file>, error out=w331:errorcluster)  [unwired: 1 in, 2 out]
                }
                n150 = xnode "Invoke Method"("FPGA VI Reference In"=w315, "error in"=w314, "Requested Depth"=w327) -> ("FPGA VI Reference Out"=w330:refnum<k20>, "error out"=w329:errorcluster)  [unwired: 1 out]
                n151 = Get Date/Time In Seconds() -> (seconds since 1Jan1904=→"Inicio pasada":timestamp)
                n152 = xnode "Invoke Method"("FPGA VI Reference In"=w330, "error in"=w329) -> ("FPGA VI Reference Out"=w324:refnum<k20>, "error out"=w323:errorcluster)
              }
              frame #1 {
                n153 = while "Data Acquisition" {
                  tunnel: w348 -> [w401]
                  shift-right: [w428] -> _
                  shift-left: u32 0 ("t") -> [w424]
                  tunnel: w346 -> [w429]
                  tunnel: w345 -> [w427]
                  shift-right: [w430] -> w350
                  shift-left: w347 -> [w421]
                  tunnel: [w425] -> w351
                  tunnel: w344 -> [w407]
                  tunnel: [w408] -> w349
                  shift-right: [w406] -> w342
                  shift-left: w343 -> [w417]
                  tunnel: w341 -> [w403]
                  i -> [w400]
                  stop <- w426 stop-if-true
                  # "Detector de presencia"
                  # "Mide el tiempo de paso del tren y con ello se puede calcular\nla velocidad la unidad"
                  n154 = xnode "Invoke Method"("FPGA VI Reference In"=w401, "error in"=w421, "Number of Elements"=w424, "Timeout (ms)"=0) -> ("FPGA VI Reference Out"=w397:refnum<k20>, "error out"=w405:errorcluster, "Data"=w420:fxp<+/-,24,4>[], "Elements Remaining"=w422:u32)
                  n155 = case "Data Ready" shown="Default" w424 {
                    tunnel: w429 -> [w450 _]
                    tunnel: [w449 u32 0 ("t")] -> w428
                    tunnel: w427 -> [w451 _]
                    tunnel: w422 -> [w448 _]
                    tunnel: w420 -> [_ w473]
                    tunnel: w417 -> [w447 w472]
                    tunnel: [w447 w474] -> w406
                    tunnel: w407 -> [w446 w471]
                    tunnel: [w446 w470] -> w408
                    frame 0 {
                      # "En este caso se compara los elementos que quedan\nen la FIFO del controlador con el tamaño dell bloque\nque aparece en el panel frontal. Si el número de \nelementos en la FIFO es mayor o igual que el tamaño\n del bloque se pasa al siguiente caso y se guardan \nlos datos en un archivo. El reloj que aparece es una\nespera para no consumir recursos."
                      n156 = Greater Or Equal?(x=w448, y=w451) -> (x >= y?=w452:bool)
                      n157 = case shown="False" w452 {
                        tunnel: [u32 0 ("Block Size") w456] -> w449
                        tunnel: [w455 0 ("t")] -> w453
                        tunnel: w450 -> [w455 _]
                        tunnel: w451 -> [_ w456]
                        frame False {
                        }
                        frame True {
                        }
                      }
                      n158 = call "WaitMinTimeBetweenCall.vi"("Minimum ms between calls"=w453) -> ()  [unwired: 2 in]
                    }
                    frame Default {
                      n159 = To Single Precision Float(number=w473) -> (single precision float=w460:sgl[])
                      n160 = Decimate 1D Array(w460) -> (w466:sgl[], w469:sgl[], w468:sgl[], w467:sgl[], w465:sgl[], w464:sgl[], w463:sgl[], w462:sgl[], w461:sgl[], w458:sgl[])
                      n161 = Build Array(w466, w469, w468, w467, w465, w464, w463, w462, w461, w458) -> (w459:sgl[][])
                      n162 = for {
                        tunnel: T6."little-endian" ("byte order (0:big-endian, network order)") -> [w483]
                        shift-right: [w477] -> w474
                        shift-left: w472 -> [w478]
                        tunnel: w459 -> [w481] mode=indexing
                        tunnel: w471 -> [w480] mode=indexing
                        tunnel: [w479] -> w470 mode=indexing
                        n163 = Write to Binary File(file (use dialog)=w480, data=w481, error in=w478, 5:FALSE ("prepend array or string size? (T)"), 9:w483) -> (refnum out=w479:refnum<file>, error out=w477:errorcluster)  [unwired: 2 out]
                      }
                    }
                  }
                  n164 = xnode "Read/Write Control"("FPGA VI Reference In"=w397, "error in"=w405) -> ("FPGA VI Reference Out"=w419:refnum<k20>, "error out"=w418:errorcluster, "Parar"=w393:bool, "Nº Ruedas 1"=→"Nº Ruedas 1":i32, "NºRuedas 2"=→"NºRuedas 2":i32)
                  "Parar" <- w393
                  n165 = case shown="True" w393 {
                    tunnel: [FALSE w441] -> w394
                    tunnel: [w432 w440] -> w411
                    tunnel: w403 -> [_ w437]
                    frame False {
                      n166 = local read "Inicio pasada"() -> (w435:timestamp)
                      n167 = Get Date/Time In Seconds() -> (seconds since 1Jan1904=w434:timestamp)
                      n168 = To Double Precision Float(number=w434) -> (double precision float=w431:dbl)
                      n169 = To Double Precision Float(number=w435) -> (double precision float=w436:dbl)
                      n170 = Subtract(x=w431, y=w436) -> (x-y=w432:dbl)
                      "Tiempo de paso (s)" <- w432
                      n171 = local write "Tiempo"(w431) -> ()
                    }
                    frame True {
                      n172 = local read "Tiempo extra al detector de paso (s)"() -> (w440:dbl)
                      n173 = local read "Tiempo"() -> (w445:dbl)
                      n174 = Get Date/Time In Seconds() -> (seconds since 1Jan1904=w442:timestamp)
                      n175 = To Double Precision Float(number=w442) -> (double precision float=w443:dbl)
                      n176 = Subtract(x=w443, y=w445) -> (x-y=w444:dbl)
                      "Tiempo extra de adquisición (s)" <- w444
                      n177 = Add(x="Tiempo de adquisicion", y=w437) -> (x+y=w438:dbl)
                      n178 = Greater?(x=w444, y=w438) -> (0:w441:bool)
                    }
                  }
                  "Fin" <- w394
                  n179 = xnode ("CheckLate")("FPGA VI Reference In"=w419, "error in"=w418) -> ("FPGA VI Reference Out"=w399:refnum<k20>, "error out"=w414:errorcluster, "Buffer Underflow"=→"Buffer Underflow":bool, "Buffer Overflow"=w402:bool)
                  "Buffer Overflow" <- w402
                  n180 = Greater?(x=w411, y=20.0) -> (0:w409:bool)
                  "Obstruido?" <- w409
                  n181 = call "ErrorOverFlow.vi"("Buffer Overflow"=w402) -> ("error out"=w412:errorcluster)
                  n182 = call "ErrorUnderFlow.vi"() -> ("error out"=w413:errorcluster)  [unwired: 1 in]
                  n183 = Merge Errors(w414, w413, w412) -> (w398:errorcluster)
                  n184 = Unbundle By Name(w406) -> ("status"=w410:bool)
                  n185 = Unbundle By Name(w398) -> ("status"=w416:bool)
                  n186 = Compound Arithmetic op=OR(w416, w394, w409, w410) -> (w426:bool)
                  "result" <- w426
                  n187 = case "Flush" shown="True" w426 {
                    tunnel: [w484 w489] -> w430
                    tunnel: [w485 w488] -> w425
                    tunnel: w399 -> [w485 w487]
                    tunnel: w398 -> [w484 w486]
                    frame False {
                    }
                    frame True {
                      n188 = xnode "Invoke Method"("FPGA VI Reference In"=w487, "error in"=w486) -> ("FPGA VI Reference Out"=w488:refnum<k20>, "error out"=w489:errorcluster)
                    }
                  }
                  "Block Size" <- w427
                  "Time to Acquire Block (ms)" <- w429
                  "Numeric 3" <- w400
                }
                n189 = disable-structure shown="Disabled" {
                  disable-tunnel: w338 -> [w356 _]
                  disable-tunnel: [w355 _] -> w337
                  frame Disabled {
                    n190 = while {
                      shift-right: [w364] -> w355
                      shift-left: w356 -> [w365]
                      shift-right: [w363] -> w354
                      shift-left: string[] [] -> [w362]
                      shift-right: [w358] -> w352
                      shift-left: i32[] [] -> [w359]
                      i -> [w360]
                      stop <- w361 stop-if-true
                      n191 = case shown="Error" w365 {
                        selector: w365 -> [w376 _]
                        tunnel: [w375 w390] -> w364
                        tunnel: [w371 string[] []] -> w363
                        tunnel: w362 -> [w370 _]
                        tunnel: w360 -> [w369 _]
                        tunnel: w359 -> [w368 _]
                        tunnel: [w367 i32[] []] -> w358
                        frame No Error {
                          n192 = call "LH6HD.vi"("error in (no error)"=w376, "Action"=enum16{"Init", "Start", "Read", "Stop", "Exit"}."Read") -> ("error out"=w375:errorcluster, "Tag"=w372:string)  [unwired: 8 in]
                          n193 = Not Equal?(x="", y=w372) -> (x != y?=w373:bool)
                          n194 = case shown="False" w373 {
                            tunnel: w372 -> [_ w385]
                            tunnel: [w379 w384] -> w371
                            tunnel: w370 -> [w379 w383]
                            tunnel: w369 -> [_ w380]
                            tunnel: w368 -> [w378 w382]
                            tunnel: [w378 w381] -> w367
                            frame False {
                            }
                            frame True {
                              n195 = Build Array (concatenate)(w383, w385) -> (w384:string[])
                              n196 = Build Array (concatenate)(w382, w380) -> (w381:i32[])
                            }
                          }
                        }
                        frame Error {
                          n197 = local read "LR6 IP address"() -> (w387:string)
                          n198 = local read "Port LR6"() -> (w388:u16)
                          n199 = call "LH6HD.vi"("DeviceAddress"=u8 0, "Reader Port"=w388, "IP Address"=w387, "Action"=enum16{"Init", "Start", "Read", "Stop", "Exit"}."Init") -> ("error out"=w390:errorcluster)  [unwired: 6 in, 1 out]
                        }
                      }
                      n200 = Wait Until Next ms Multiple(millisecond multiple=u32 500) -> ()  [unwired: 1 out]
                      n201 = local read "result"() -> (w361:bool)
                      "it-LR6" <- w360
                    }
                    "TAGs LR6" <- w354
                    "it-read-LR6" <- w352
                  }
                  frame Enabled {
                  }
                }
                n202 = Merge Errors(w337) -> (w339:errorcluster)
              }
              frame #2 {
                (unwired) u32 1000 ("Number of Elements")
                n203 = Array Size(array=w510) -> (size(s)=w508:i32)
                n204 = Decrement(x=w508) -> (x-1=w509:i32)
                n205 = local read "Puerto RFID"() -> (w525:u16)
                n206 = call "LH6HD.vi"("error in (no error)"=w503, "Action"=enum16{"Init", "Start", "Read", "Stop", "Exit"}."Stop") -> ("error out"=w502:errorcluster)  [unwired: 8 in, 1 out]
                n207 = local read "RFID_Error"() -> (w536:errorcluster)
                n208 = local read "IP RFID"() -> (w507:string)
                n209 = local read "RFID_ID"() -> (w535:refnum<k5>)
                n210 = Index Array(array=w510, index=w509) -> (element=w518:refnum<file>)
                n211 = local write "result"(FALSE ("result")) -> ()
                n212 = xnode "Read/Write Control"("FPGA VI Reference In"=w495, "error in"=w494) -> ("FPGA VI Reference Out"=w493:refnum<k20>, "error out"=w492:errorcluster, "Direccion 0?"=→"Direccion 0?":bool)
                n213 = local write "RFID_LR6_Error"(w502) -> ()
                n214 = disable-structure shown="Enabled" {
                  disable-tunnel: [w566 _] -> w537
                  disable-tunnel: w536 -> [w565 w568]
                  disable-tunnel: w535 -> [w564 _]
                  disable-tunnel: [w563 _] -> w534
                  disable-tunnel: [w562 w568] -> w529
                  disable-tunnel: w525 -> [w561 _]
                  disable-tunnel: w507 -> [w560 _]
                  disable-tunnel: [w559 "TAGs HEX 2"] -> w500
                  frame Enabled {
                    n215 = call "RFID_28_03_12.vi"("BYTES TO READ"=2000, "TIMEOUT"=25, "RFID_Error"=w565, "Puerto RFID"=w561, "IP RFID"=w560, "RFID ID"=w564) -> ("RFID Error"=w562:errorcluster, "connection ID out"=w563:refnum<k5>, "TAGs HEX"=w559:string[], "Unidad"=w566:u32)  [unwired: 1 in]
                    "RFID_Error 2" <- w565
                  }
                  frame Disabled {
                  }
                }
                "TAGs HEX" <- w500
                n216 = local read "TAGs LR6"() -> (w501:string[])
                n217 = Index Array(array=w500) -> (element=w499:string)  [unwired: 1 in]
                n218 = Not Equal?(x=w499, y="" ("delimiter (\\t)")) -> (x != y?=w497:bool)
                "Plataformas?" <- w497
                n219 = case shown="True" w497 {
                  tunnel: w501 -> [w550 w551]
                  tunnel: [w550 w553] -> w505
                  tunnel: w500 -> [_ w552]
                  frame False {
                  }
                  frame True {
                    n220 = call "Union_TAGs_RFIDs.vi"("TAGs LR6"=w551, "TAGs HEX"=w552) -> ("TAGs"=w553:string[])
                  }
                }
                "TAGs" <- w505
                n221 = local read "Tiempo de paso (s)"() -> (w532:dbl)
                n222 = local read "Nombre de archivo"() -> (w517:path[])
                n223 = xnode "Read/Write Control"("FPGA VI Reference In"=w493, "error in"=w492) -> ("FPGA VI Reference Out"=w539:refnum<k20>, "error out"=w538:errorcluster, "Chassis Temperature"=w548:i16)
                n224 = Multiply(x=w532, y=1000.0) -> (x*y=w530:dbl)
                n225 = for {
                  shift-right: [w571] -> w523
                  shift-left: string[] [] -> [w570]
                  tunnel: w505 -> [w569] mode=indexing
                  n226 = Insert Into Array(array=w570, new element=w569) -> (w571:string[])  [unwired: 1 in]
                }
                n227 = Divide(x=w548, y=4.0) -> (x/y=w549:dbl)
                "Temperatura (ºC)" <- w549
                n228 = Build Array(w549, w530, w537) -> (w543:dbl[])
                n229 = local write "RFID_ID"(w534) -> ()
                n230 = local write "RFID_Error"(w529) -> ()
                n231 = Delete From Array(array=w517) -> (deleted portion=w516:path)  [unwired: 2 in, 1 out]
                n232 = To Single Precision Float(number=w543) -> (single precision float=w546:sgl[])
                n233 = xnode "Read/Write Control"("FPGA VI Reference In"=w539, "error in"=w538, "Stop"=TRUE ("stop")) -> ("FPGA VI Reference Out"=w520:refnum<k20>, "error out"=w519:errorcluster)
                n234 = Path To String(path=w516) -> (string=w522:string)
                n235 = Write to Binary File(file (use dialog)=w518, data=w546, error in=w542, 5:FALSE ("prepend array or string size? (T)"), 9:T6."little-endian" ("byte order (0:big-endian, network order)")) -> (error out=w515:errorcluster)  [unwired: 3 out]
                n236 = Build Array (concatenate)(w522, w523) -> (w490:string[])
                n237 = local read "TAGS leidos"() -> (w511:path)
                n238 = local read "Obstruido?"() -> (w533:bool)
                n239 = for {
                  shift-right: [w556] -> w526
                  shift-left: w515 -> [w555]
                  tunnel: w510 -> [w554] mode=indexing
                  n240 = Close File(refnum=w554, error in=w555) -> (error out=w556:errorcluster)  [unwired: 1 out]
                }
                n241 = xnode "Invoke Method"("FPGA VI Reference In"=w520, "error in"=w519) -> ("FPGA VI Reference Out"=w528:refnum<k20>, "error out"=w527:errorcluster)
                n242 = call-poly <vilib>:"Write Delimited Spreadsheet.vi"("file path (dialog if empty)"=w511, "1D data"=w490, "append to file? (F)"=FALSE ("transpose? (no:F)"), "transpose? (F)"=TRUE ("append to file? (new file:F)"), "delimiter (\\t)"=";" ("delimiter (\\t)")) -> ()  [unwired: 9 in, 2 out]
                n243 = Select(t="Escape", s=w533, f="Procesado") -> (s? t:f=w540:string)
              }
            }
            n244 = Random Number (0-1)() -> (number: 0 to 1=w278:dbl)
            n245 = Multiply(x=2, y=w278) -> (x*y=w276:dbl)
            n246 = Unbundle By Name(w294) -> ("status"=w283:bool)
            n247 = Unbundle By Name(w292) -> ("status"=w284:bool)
            n248 = Merge Errors(w292) -> (w291:errorcluster)
            n249 = Compound Arithmetic op=OR(w283, w284) -> (w281:bool)
            n250 = Select(t="TEST", s=w281, f=w282) -> (s? t:f=w279:string)
          }
          frame "Procesado" {
            n251 = flat-sequence {
              tunnel: w572 -> [w594]
              tunnel: [w597] -> w575
              tunnel: [w782] -> w585
              tunnel: w575 -> [w782]
              frame #0 {
                n252 = flat-sequence {
                  tunnel: [w656] -> w596
                  tunnel: [w640] -> w595
                  tunnel: w594 -> [_]
                  tunnel: [w643] -> w593
                  tunnel: [w629] -> w590
                  tunnel: [w642] -> w592
                  tunnel: [w628] -> w591
                  frame #0 {
                    (unwired) 3 ("Número de ejes detectados")
                    (unwired) string[] ["S200"] ("Series_flota1")
                    (unwired) i32[] [28] ("Ejes_UT")
                    (unwired) path "c:/0002_2010-05-08_08-07-07.bin" ("Nombre de archivo")
                    # "UNIR AL\nSELECTOR"
                    # "Unidad 514"
                    # "Señal del inductivo"
                    # "Estos indicadores sirven para controlar que no se sature la memoria"
                    # "Distancia de\nla unidad"
                    n253 = disable-structure shown="Disabled" {
                      disable-tunnel: [w662 w664] -> w617
                      frame Enabled {
                        n254 = local read "Nombre de archivo"() -> (w662:path[])
                      }
                      frame Disabled {
                        n255 = Delete From Array(array="Array", index (col)="Índice de los archivos seleccionados") -> (deleted portion=w664:path[])  [unwired: 2 in, 1 out]
                      }
                    }
                    n256 = disable-structure shown="Enabled" {
                      disable-tunnel: [w660 string[] ["13690667", "6583", "6584"] ("Series_flota1")] -> w633
                      frame Disabled {
                        n257 = local read "TAGs"() -> (w660:string[])
                      }
                      frame Enabled {
                      }
                    }
                    n258 = local read "Tabla_flota"() -> (w639:string[][])
                    n259 = call "Series_ejes_flota.vi"("Tabla_flota"=w639, "Tags"=w633) -> ("Nº Ejes"=w622:i32[], "Series del convoy"=w632:string[])  [unwired: 2 in, 1 out]
                    n260 = local read "Puntos medios de las ventanas"() -> (w641:dbl[][])
                    n261 = Array Size(array=w617) -> (size(s)=w649:i32)
                    n262 = Add Array Elements(numeric array=w622) -> (sum=w621:i32)
                    "Ejes_convoy" <- w621
                    n263 = Subtract(x=w649, y=2 ("length")) -> (x-y=w651:i32)
                    n264 = Array Size(array=w632) -> (size(s)=→"Nº UTs":i32)
                    n265 = local read "Direccion 0?"() -> (w616:bool)
                    n266 = Delete From Array(array=w617, length=2, index=w651) -> (deleted portion=w613:path[], array with subset deleted=w642:path[])
                    n267 = Index Array(array=w613) -> (element #1=w599:path, element #2=w598:path)  [unwired: 2 in]
                    n268 = case shown="True" "Señal digital?" {
                      tunnel: [sgl[] [5.23] ("x*y") w669] -> _
                      frame False {
                      }
                      frame True {
                        n269 = Multiply(x=sgl 10.0, y="x*y") -> (x*y=w669:dbl[])
                      }
                    }
                    n270 = Select(t=w599, s=w616, f=w598) -> ()  [unwired: 1 out]
                    n271 = Read from Binary File(5:sgl 0.0, 9:T6."little-endian" ("byte order (0:big-endian, network order)"), 10:-1 ("count (1)"), 11:w599) -> (0:w647:errorcluster, 2:w615:sgl[], 3:w648:refnum<file>)  [unwired: 1 in, 2 out]
                    n272 = local read "Series_flota"() -> (w638:string[])
                    n273 = Close File(refnum=w648, error in=w647) -> (error out=w643:errorcluster)  [unwired: 1 out]
                    n274 = Read from Binary File(5:sgl 0.0, 9:T6."little-endian" ("byte order (0:big-endian, network order)"), 10:-1 ("count (1)"), 11:w598) -> (0:w611:errorcluster, 2:w603:sgl[], 3:w612:refnum<file>)  [unwired: 1 in, 2 out]
                    n275 = Array Size(array=w615) -> (size(s)=w637:i32)
                    n276 = Close File(refnum=w612, error in=w611) -> ()  [unwired: 2 out]
                    n277 = Subtract(x=w637, y=3 ("length")) -> (x-y=w635:i32)
                    n278 = Array Size(array=w603) -> (size(s)=w607:i32)
                    n279 = Delete From Array(array=w615, length=3, index=w635) -> (array with subset deleted=w601:sgl[])  [unwired: 1 out]
                    n280 = call "Distancias_ejes_convoy.vi"("Series_flota1"=w632, "Ejes_UT"=w622, "Puntos medios de las ventanas"=w641, "Series_flota"=w638) -> ("Distancias_entre_ejes_convoy"=w640:dbl[])  [unwired: 1 in]
                    n281 = Subtract(x=w607, y=3 ("length")) -> (x-y=w605:i32)
                    n282 = call "Puntos medio de pulso.vi"("DI Inductivo"=w601) -> ("Puntos"=w656:sgl[], "Número de ejes"=w618:i32)  [unwired: 1 in]
                    "Número de ejes detectados" <- w618
                    n283 = Delete From Array(array=w603, length=3, index=w605) -> (array with subset deleted=w602:sgl[])  [unwired: 1 out]
                    n284 = Decrement(x=w618) -> (x-1=w655:i32)
                    n285 = local read "Tiempo de paso (s)"() -> (w654:dbl)
                    n286 = Build Array(w601, w602) -> (→"Waveform Graph":sgl[][])
                    n287 = local read "TAGs"() -> (w627:string[])
                    n288 = local read "it-LR6"() -> (w624:i32)
                    n289 = local read "it-read-LR6"() -> (w625:i32[])
                    n290 = local read "TAGs LR6"() -> (w626:string[])
                    n291 = local read "Plataformas?"() -> (w623:bool)
                    n292 = call "Calculo_Velocidad.vi"("Tiempo de paso (s)"=w654, "Ejes"=w655, "Puntos iniciales de las ventanas"=w640) -> ("V (m/s)"=→"V (m/s)":dbl, "Longitud de la unidad"=→"Longitud de la unidad":dbl)
                    n293 = call "TAGs_AURAwheel.vi"("Nº Ejes"=w622, "TAGs"=w627, "Ejes_convoy"=w621, "it-LR6"=w624, "TAGs LR6"=w626, "it-read-LR6"=w625, "Plataformas?"=w623) -> ("TAGS_AURA"=→"TAGs_AURAwheel":string[][])  [unwired: 1 in]
                    n294 = call "Comprobación Señal digital (SubVI).vi"("Inductivo"=w601) -> ("Señal digital?"=w630:bool)
                    n295 = Get Volume Info(11:path "c:/" ("path")) -> (1:→"Disco Duro Disponible (bytes)":i64)  [unwired: 1 in, 5 out]
                    n296 = Equal?(x=w618, y=w618) -> (x = y?=w628:bool)
                    n297 = And(x=w628, y=w630) -> (x .and. y?=w629:bool)
                    "Nº Ejes" <- i32[] [3, 3] ("Nº Ejes")
                  }
                }
                n298 = case shown="False" w590 {
                  tunnel: w593 -> [w672 w702]
                  tunnel: [w672 w701] -> w597
                  tunnel: w596 -> [_ w706]
                  tunnel: w595 -> [_ w704]
                  tunnel: w592 -> [_ w705]
                  tunnel: w591 -> [w670 _]
                  frame False {
                    n299 = local read "Nombre de archivo"() -> (w671:path[])
                    n300 = for {
                      tunnel: w671 -> [w674] mode=indexing
                      tunnel: w670 -> [w673]
                      n301 = flat-sequence {
                        tunnel: w674 -> [w684]
                        tunnel: [w684] -> w677
                        tunnel: [w683] -> w676
                        tunnel: w673 -> [w682]
                        tunnel: w677 -> [w690]
                        tunnel: [w689] -> w675
                        tunnel: w676 -> [w689]
                        tunnel: w675 -> [w692]
                        frame #0 {
                          w683 = path "c:/Est_Adq.csv" ("file path (use dialog)")
                          n302 = Path To String(path=w684) -> (string=w685:string)
                          n303 = Select(t="Nº Ejes detectados WS diferente a Nº Ejes TAGs" ("delimiter (\\t)"), s=w682, f="La señal del inductivo no es digital" ("delimiter (\\t)")) -> (s? t:f=w679:string)
                          n304 = Build Array(w685, w679) -> (w678:string[])
                          n305 = call-poly <vilib>:"Write Delimited Spreadsheet.vi"("file path (dialog if empty)"=w683, "1D data"=w678, "append to file? (F)"=FALSE ("transpose? (no:F)"), "transpose? (F)"=TRUE ("append to file? (new file:F)"), "delimiter (\\t)"=";" ("delimiter (\\t)")) -> ()  [unwired: 9 in, 2 out]
                        }
                        frame #1 {
                          n306 = disable-structure shown="Enabled" {
                            disable-tunnel: w690 -> [w691 _]
                            frame Enabled {
                              n307 = Delete(path (use dialog)=w691) -> ()  [unwired: 1 in, 6 out]
                            }
                            frame Disabled {
                            }
                          }
                        }
                        frame #2 {
                          n308 = File/Directory Info(path=w692) -> (size=w695:i64)  [unwired: 1 in, 6 out]
                          n309 = Greater?(x=w695, y=i64 1000000) -> (0:w693:bool)
                          n310 = case shown="True" w693 {
                            tunnel: w692 -> [_ w696]
                            frame False {
                            }
                            frame True {
                              n311 = Delete(path (use dialog)=w696) -> ()  [unwired: 4 in, 3 out]
                            }
                          }
                        }
                      }
                    }
                  }
                  frame True {
                    n312 = flat-sequence {
                      tunnel: w706 -> [w772]
                      tunnel: w705 -> [w768]
                      tunnel: w704 -> [w773]
                      tunnel: [w766] -> w703
                      frame #0 {
                        # "Entrada:\n- dt RMS\n- Paths\n- Param_acelerometros (sensivity)\n- Parm_filtro\n- Puntos ventana\n- error\n- Frecuencia\n- Velocidad ejes\n- Punto medio paso rueda (p)"
                        # "SALIDA \n\nMáximos por rueda inductivo"
                        # "ENTRADA \nNúmero de ejes\nDistancia de acelerómetros\nDistancias del centro de las ruedas\nPuntos medios de las ruedas (INDUCTIVO)\nFrecuencia\ndt RMS\nDistancias generales\nAceleraciones"
                        # "8 acelerómetros"
                        # "Velocidad"
                        n313 = local read "Frecuencia de muestreo (Hz)"() -> (w771:dbl)
                        n314 = local read "Distancia de acelerómetros"() -> (w774:dbl[])
                        n315 = local read "Parámetros acelerómetros"() -> (w765:dbl[])
                        n316 = local read "Número de ejes detectados"() -> (w764:i32)
                        n317 = local read "Distancias generales"() -> (w769:dbl[])
                        n318 = local read "dt RMS"() -> (w770:dbl)
                        n319 = call "Procesado_aRMS_BIdirecc.vi"("Paths_canales_aRMS"=w768, "Distancias generales (m)"=w769, "Distancias\nacelerometros"=w774, "Ejes Procesados"=w764, "Distancias centrales de las ruedas\n               configuración (m)"=w773, "Frecuencia de muestreo"=w771, "Parámetros acelerómetros"=w765, "dt RMS 2"=w770, "Puntos"=w772) -> ("Max RMS Ruedas"=w767:dbl[][])  [unwired: 1 in]
                        n320 = Transpose 2D Array(2D array=w767) -> (transposed array=w766:dbl[][])
                        "Max RMS Ruedas" <- w766
                      }
                    }
                    n321 = disable-structure shown="Disabled" {
                      disable-tunnel: [w762 TRUE ("Use Aura?")] -> w700
                      frame Disabled {
                        n322 = local read "Use Aura?"() -> (w762:bool)
                      }
                      frame Enabled {
                      }
                    }
                    n323 = local read "TAGs_AURAwheel"() -> (w698:string[][])
                    n324 = local read "Nº Ejes"() -> (w697:i32[])
                    n325 = for {
                      tunnel: w700 -> [w711]
                      tunnel: [w710] -> w699 mode=indexing
                      tunnel: w698 -> [w709] mode=indexing
                      shift-right: [w708] -> _
                      shift-left: w703 -> [w712]
                      tunnel: w697 -> [w707] mode=indexing
                      # "dev.api.aurawheel.com"
                      n326 = case shown="True" w711 {
                        tunnel: w712 -> [w713 w719]
                        tunnel: [errorcluster {"status"=FALSE, "code"=0, "source"=""} ("error out") w731] -> w710
                        tunnel: w709 -> [_ w720]
                        tunnel: [w713 w718] -> w708
                        tunnel: w707 -> [_ w716]
                        frame False {
                        }
                        frame True {
                          (unwired) "http://dev.api.aurawheel.com/services/wrd/upload"
                          (unwired) "tagMexFin"
                          (unwired) "tagMexInit"
                          (unwired) "tag2"
                          (unwired) "tag1"
                          w735 = cluster{"status":string} {"status"=""}
                          n327 = local read "TAGs"() -> (w726:string[])
                          n328 = local read "Parametros AuraWheel"() -> (w760:string[])
                          n329 = Delete From Array(array=w719, length=w716, index (row)=0) -> (deleted portion=w715:dbl[][], array with subset deleted=w718:dbl[][])  [unwired: 1 in]
                          n330 = Get Date/Time In Seconds() -> (seconds since 1Jan1904=w756:timestamp)
                          n331 = Delete From Array(array=w726, length=2, index=0) -> ()  [unwired: 2 out]
                          n332 = Format Date/Time String(time format string (%c)="%H:%M:%S%3u", seconds (now)=w756) -> (date/time string=w754:string)  [unwired: 1 in]
                          n333 = Get Date/Time In Seconds() -> (seconds since 1Jan1904=w730:timestamp)
                          n334 = Scan From String(format string="%d:%d:%f", input string=w754) -> (output 1=w751:i32, output 2=w750:i32, output 3=w748:dbl)  [unwired: 5 in, 3 out]
                          n335 = local read "Temperatura (ºC)"() -> (w728:dbl)
                          n336 = disable-structure shown="Enabled" {
                            disable-tunnel: [_ 60.0 ("p_sp")] -> w727
                            frame Disabled {
                              n337 = local read "V (m/s)"() -> ()  [unwired: 1 out]
                            }
                            frame Enabled {
                            }
                          }
                          n338 = Multiply(x=w748, y=1000.0) -> (x*y=w744:dbl)
                          n339 = call "Time_to_ms.vi"("seconds since 1Jan1904"=w730) -> ("Numeric"=w729:dbl)  [unwired: 1 in]
                          n340 = Multiply(x=w750, y=60000) -> (x*y=w745:i32)
                          n341 = Multiply(x=3600000, y=w751) -> (x*y=w746:i32)
                          n342 = Index Array(array=w760) -> ()  [unwired: 3 in, 3 out]
                          n343 = call "aw_WRDCluster_8acel.vi"("Array TAGs"=w720, "Max RMS Ruedas"=w715, "TimeStamp"=w729, "p_sp"=w727, "p_tp"=w728) -> ("JSON cluster"=w757:T8)  [unwired: 1 in]
                          n344 = Compound Arithmetic op=ADD(w746, w745, w744) -> (w743:dbl)
                          n345 = To Variant(anything=w757) -> (Variant=w740:variant)
                          n346 = To Unsigned Long Integer(number=w743) -> (unsigned 32bit integer=w742:u32)
                          n347 = call "gjson_Create.vi"("JSON Object in"=w740) -> ("error out"=w738:errorcluster, "JSON String Out"=w739:string)  [unwired: 9 in]
                          n348 = Number To Decimal String(number=w742) -> (decimal integer string=w741:string)  [unwired: 1 in]
                          n349 = To Variant(anything=w735) -> (Variant=w734:variant)
                          n350 = call "aw_SendData.vi"("pwd"="wrd", "x-nem-datetime"=w741, "User"="User", "error in"=w738, "JSON Object"=w739, "URL"="http://api.aurawheel.dev/services/wrd/upload") -> ("error out"=w736:errorcluster, "Response JSON"=w737:string, "Response headers"=→"Response headers":string)  [unwired: 3 in]
                          n351 = call "gjson_Parse.vi"("error in"=w736, "JSON String In"=w737, "JSON Cluster"=w734) -> ("error out"=w732:errorcluster, "JSON Cluster Out"=w733:variant)  [unwired: 7 in]
                          n352 = Variant To Data(error in=w732, type=w735, Variant=w733) -> (data=→"data":cluster{"status":string}, error out=w731:errorcluster)
                          "error AURA" <- w731
                        }
                      }
                    }
                    n353 = Merge Errors(w699, w702) -> (w701:errorcluster)
                  }
                }
              }
              frame #1 {
                n354 = local read "TAGS leidos"() -> (w778:path)
                n355 = local read "Nombre de archivo"() -> (w775:path[])
                n356 = File/Directory Info(path=w778) -> (size=w781:i64)  [unwired: 1 in, 6 out]
                n357 = local read "Path TEST"() -> (w777:path)
                n358 = disable-structure shown="Disabled" {
                  frame Disabled {
                    n359 = call "Borrar_carpeta.vi"("Nº Archivos Max"=1000, "Path Carpeta"=path "c:/Trenes") -> ()  [unwired: 1 in]
                  }
                  frame Enabled {
                  }
                }
                n360 = Greater?(x=w781, y=i64 1000000) -> (0:w779:bool)
                n361 = case shown="True" w779 {
                  tunnel: w778 -> [_ w785]
                  frame False {
                  }
                  frame True {
                    n362 = Delete(path (use dialog)=w785) -> ()  [unwired: 4 in, 3 out]
                  }
                }
                n363 = call "Borrar_carpeta.vi"("Nº Archivos Max"=i64 250 ("y"), "Path Carpeta"=w777) -> ()  [unwired: 1 in]
                n364 = call "Retrieve_memory_3_folders.vi"() -> ()  [unwired: 12 in]
                n365 = call "Comprimir_a_1_archivo.vi"("Acel_paths"=w775) -> ()  [unwired: 1 out]
              }
            }
            n366 = disable-structure shown="Disabled" {
              disable-tunnel: [w589 _] -> w573
              frame Disabled {
                n367 = local read "IP synchr"() -> (w588:string)
                n368 = call "Synchronization.vi"("Time Server\nIP Address"=w588) -> ("error out"=w589:errorcluster)
              }
              frame Enabled {
              }
            }
            n369 = local read "RFID_Error"() -> (w576:errorcluster)
            n370 = Merge Errors(w585) -> (w577:errorcluster)
            n371 = Merge Errors(w574, w573, w576, w577) -> (w586:errorcluster)
            n372 = Unbundle By Name(w586) -> ("status"=w580:bool)
            n373 = Select(t="Descarga datos", s=FALSE, f="Espera") -> (s? t:f=w582:string)
            n374 = Select(t="TEST", s=w580, f=w582) -> (s? t:f=w579:string)
          }
          frame "TEST" {
            n375 = flat-sequence {
              tunnel: [w796] -> w791
              tunnel: w790 -> [w811]
              tunnel: w788 -> [w810]
              tunnel: [w809] -> w787
              tunnel: [w792] -> w786
              frame #0 {
                n376 = Get Date/Time In Seconds() -> (seconds since 1Jan1904=w803:timestamp)
                n377 = local read "Ultimo TEST"() -> (w804:timestamp)
                n378 = To Double Precision Float(number=w803) -> (double precision float=w805:dbl)
                n379 = Subtract(x=w805, y=3600.0) -> (x-y=w807:dbl)
                n380 = To Time Stamp(1:w807) -> (0:w808:timestamp)
                n381 = In Range and Coerce(upper limit=w803, x=w804, lower limit=w808) -> (In Range?=w802:bool)  [unwired: 1 out]
                n382 = case shown="False" w802 {
                  tunnel: w811 -> [w841 _]
                  tunnel: w810 -> [w816 w847]
                  tunnel: [w826 errorcluster {"status"=FALSE, "code"=0, "source"=""} ("error out")] -> w809
                  tunnel: [w816 w847] -> w792
                  frame False {
                    n383 = local read "Obstruido?"() -> (w818:bool)
                    n384 = case shown="True" w818 {
                      selector: w818 -> [_ w843]
                      tunnel: ["\r" w844] -> w815
                      frame False {
                      }
                      frame True {
                        n385 = call "ErrorObstruccion.vi"("Buffer Overflow"=w843) -> ("error out"=w846:errorcluster)
                        n386 = call "Error.vi"("Error con..."="Warning:", "error comunicacion 2"=w846) -> ("String"=w844:string)
                      }
                    }
                    n387 = local read "Aviso no detección"() -> (w824:string)
                    n388 = local read "Aviso temperatura"() -> (w823:string)
                    n389 = local read "RFID_Error"() -> (w820:errorcluster)
                    n390 = local read "RFID_LR6_Error"() -> (w813:errorcluster)
                    n391 = local read "DC OK"() -> (w822:string)
                    n392 = local read "Fallo sensores"() -> (w817:string)
                    n393 = call "Cabecera.vi"() -> ("String"=w839:string)
                    n394 = call "Adquisicion.vi"("Aviso no detección"=w824) -> ("String"=w838:string)
                    n395 = call "Temperatura.vi"("Aviso temperatura"=w823) -> ("String"=w837:string)
                    n396 = call "Fuente.vi"("DC OK"=w822) -> ("String"=w836:string)
                    n397 = call "FPGA.vi"("error out"=w816) -> ("String"=w835:string)
                    n398 = call "Escritura.vi"("error out"=w841) -> ("String"=w834:string)
                    n399 = call "Error.vi"("Error con..."="Error con el lecto RFID NEM", "error comunicacion 2"=w820) -> ("String"=w819:string)
                    n400 = call "Error.vi"("Error con..."="Error con el lecto RFID LR6-HD", "error comunicacion 2"=w813) -> ("String"=w812:string)
                    n401 = Concatenate Strings(w839, w838, w837, w836, w835, w834, w817, w819, w812, w815) -> (w840:string)
                    n402 = call "STRINGhorafechA(SubVI).vi"() -> ("STRINGhora_fecha"=w833:string)
                    n403 = Concatenate Strings(w833, ".txt" ("string")) -> (w829:string)
                    n404 = Get Date/Time In Seconds() -> (seconds since 1Jan1904=→"Ultimo TEST":timestamp)
                    n405 = Build Array("c", "TEST" ("element"), w829) -> (w831:string[])
                    n406 = Array of Strings to Path(0:w831) -> (2:w827:path)  [unwired: 1 out]
                    n407 = Write to Text File(file (use dialog)=w827, text=w840) -> (error out=w826:errorcluster)  [unwired: 1 in, 3 out]
                  }
                  frame True {
                  }
                }
                n408 = local read "Fallo fotocelula"() -> (w795:bool)
                n409 = Unbundle By Name(w792) -> ("status"=w793:bool)
                n410 = local read "T fuera rango"() -> (w801:bool)
                n411 = Compound Arithmetic op=OR(w793, w795) -> (w794:bool)
                n412 = local write "Reset del controlador"(w794) -> ()
                n413 = Select(t="Escape", s=w801, f="Espera") -> (s? t:f=w798:string)
                n414 = Select(t="Configuracion", s=w794, f=w798) -> (s? t:f=w796:string)
              }
            }
          }
          frame "Escape" {
            n415 = while {
              tunnel: w852 -> [w868]
              tunnel: [w867] -> w853
              shift-right: [w866] -> w850
              shift-left: w849 -> [w855]
              stop <- w858 stop-if-true
              # "Espera hasta que el detector de\npresencia se desactive"
              n416 = Wait (ms)(milliseconds to wait=u32 3000) -> ()  [unwired: 1 out]
              n417 = xnode "Read/Write Control"("FPGA VI Reference In"=w868, "error in"=w855) -> ("FPGA VI Reference Out"=w867:refnum<k20>, "error out"=w866:errorcluster, "Detector de presencia"=w864:bool, "Chassis Temperature"=w859:i16)
              n418 = Divide(x=w859, y=4.0) -> (x/y=w860:dbl)
              n419 = In Range and Coerce(upper limit=55.0, x=w860, lower limit=0.0) -> (In Range?=w856:bool)  [unwired: 1 out]
              n420 = Not(x=w864) -> (.not. x?=w857:bool)
              n421 = And(x=w857, y=w856) -> (x .and. y?=w858:bool)
            }
          }
        }
        "Estado" <- w64
        "error manipulacion archivos" <- w66
        n422 = local read "Parar la aplicación"() -> (w63:bool)
      }
      n423 = xnode "Close FPGA VI Reference"("FPGA VI Reference In"=w56, "error in"=w55) -> ("error out"=→"error FPGA":errorcluster)
    }
    frame #3 {
      n424 = local read "RFID_ID"() -> (w871:refnum<k5>)
      n425 = call "LH6HD.vi"("Action"=enum16{"Init", "Start", "Read", "Stop", "Exit"}."Stop") -> ("error out"=→"RFID_LR6_Error":errorcluster)  [unwired: 9 in, 1 out]
      n426 = TCP Close Connection(connection ID=w871) -> (error out=→"RFID_Error":errorcluster)  [unwired: 1 in, 2 out]
    }
  }
